vi "Autonomous Independent.vi"() -> ()   [LabVIEW 2020]
doc: "This VI is called when autonomous begins, and will automatically be terminated when autonomous ends. You can carry out timed or sensor driven robot movement independently without needing to return to the caller."
uses:
  <vilib>/Rock Robotics/WPI/Solenoid/WPI_SolenoidValue.ctl
  <vilib>/Rock Robotics/WPI/Utilities/WPI_GetSetVariantRefNum.vi
  <vilib>/Rock Robotics/Network Tables/NT Read String.vi
  <vilib>/Rock Robotics/Network Tables/NT Write Numeric Array.vi
  <vilib>/Rock Robotics/WPI/Solenoid/WPI_SolenoidSetEnum.vi
panel:
  out "substring":string
  in  "Array of robot movements 2":T1(array[cluster])=[{"X Joystick Value"=0.39393939393939403, "Y Joystick Value"=0.0, "Delay (sec)"=1.0, "Movement Name"="turn"}, {"X Joystick Value"=-0.3737373737373737, "Y Joystick Value"=0.0, "Delay (sec)"=1.0, "Movement Name"="turn back"}] {"Y Joystick Value" scale=1.0..-1.0; "X Joystick Value" scale=-1.0..1.0}
  # "Be sure to right-click and choose Data Operations>>Make Current Value default if you want to save the array values with the VI"
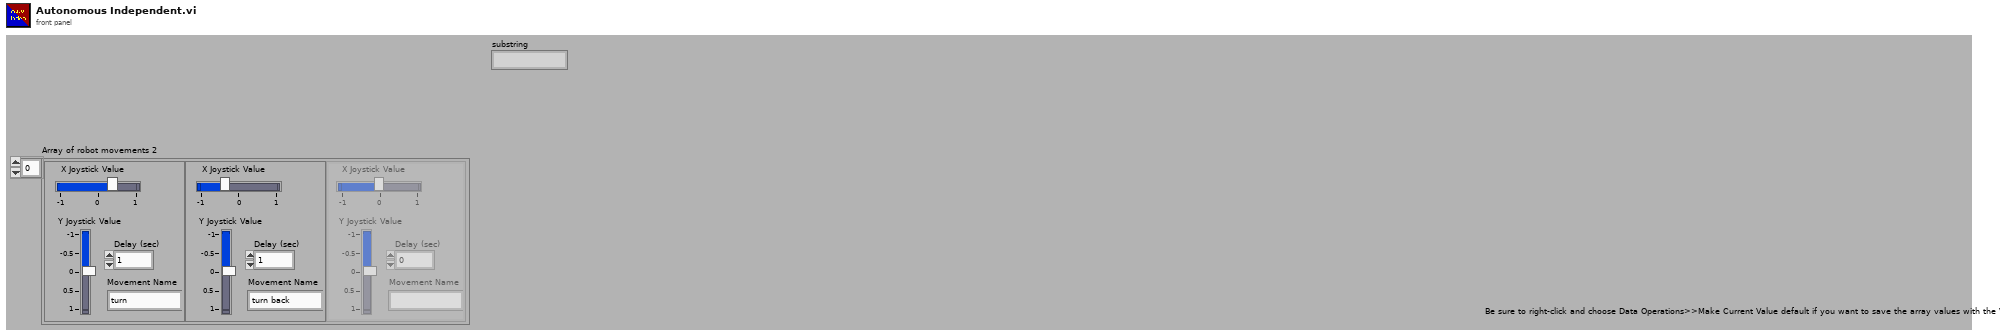
[diagram p1: front panel]
types:
  T1 = cluster{"X Joystick Value":dbl, "Y Joystick Value":dbl, "Delay (sec)":dbl, "Movement Name":string}[]
  T2 = typedef "WPI_JoystickDevRef.ctl" = cluster{"Device":T3}
  T3 = typedef "WPI_JoystickDeviceEnum.ctl" = enum16{"USB 0", "USB 1", "USB 2", "USB 3", "USB 4", "USB 5"}
  T4 = typedef "WPI_SolenoidValue.ctl" = enum16{"Off", "On", "Forward", "Reverse"}
  T5 = typedef "WPI_RobotDriveDevRef.ctl" = cluster{"DevStatus":errorcluster, "Motors[]":T6[], "Square Inputs":bool, "Max Output":dbl}
  T6 = typedef "WPI_MotorControlDeviceRef.ctl" = cluster{"DeviceStatus":errorcluster, "Type":T7, "PWM":cluster{"PWM Channel":T8, "DeadBand":T9}, "CAN":cluster{"Device Number":u8, "SetOutput VI Ref":variant, "GetOutput VI Ref":variant, "Enable VI Ref":variant, "Disable VI Ref":variant, "Data":variant}, "Invert":bool, "DIO PWM":cluster{"PWM \"Enable\" Channel":T8, "DIOChannel":T10, "PWM Rate":dbl}}
  T7 = typedef "WPI_MotorControlType.ctl" = enum16{"PWM", "CAN", "DIO PWM"}
  T8 = typedef "FPGA_DIOPWMChannel.ctl" = enum8{"PWM 0", "PWM 1", "PWM 2", "PWM 3", "PWM 4", "PWM 5", "PWM 6", "PWM 7", "PWM 8", "PWM 9", "PWM MXP 0", "PWM MXP 1", "PWM MXP 2", "PWM MXP 3", "PWM MXP 4", "PWM MXP 5", "PWM MXP 6", "PWM MXP 7", "PWM MXP 8", "PWM MXP 9", "Invalid"}
  T9 = typedef "WPI_PWMDeadband.ctl" = cluster{"Name":string, "maxPositivePwm":i32, "minPositivePwm":i32, "centerPwm":i32, "maxNegativePwm":i32, "minNegativePwm":i32, "angularRange":u16}
  T10 = typedef "FPGA_DIOChannel.ctl" = enum8{"DIO 0", "DIO 1", "DIO 2", "DIO 3", "DIO 4", "DIO 5", "DIO 6", "DIO 7", "DIO 8", "DIO 9", "DIO MXP 0", "DIO MXP 1", "DIO MXP 2", "DIO MXP 3", "DIO MXP 4", "DIO MXP 5", "DIO MXP 6", "DIO MXP 7", "DIO MXP 8", "DIO MXP 9", "DIO MXP 10", "DIO MXP 11", "DIO MXP 12", "DIO MXP 13", "DIO MXP 14", "DIO MXP 15", "SPI Port CS1", "SPI Port CS2", "SPI Port CS3", "SPI Port MISO", "SPI Port MOSI", "Invalid"}
  T11 = typedef "WPI_SolenoidDevRef.ctl" = cluster{"DevStatus":errorcluster, "Pneumatics Control Module":u8, "Forward Solenoid Channel":T12, "Reverse Solenoid Channel":T12}
  T12 = typedef "WPI_SolenoidChannel.ctl" = enum8{"Solenoid 0", "Solenoid 1", "Solenoid 2", "Solenoid 3", "Solenoid 4", "Solenoid 5", "Solenoid 6", "Solenoid 7", "Solenoid 8", "Solenoid 9", "Solenoid 10", "Solenoid 11", "Solenoid 12", "Solenoid 13", "Solenoid 14", "Solenoid 15", "Invalid"}
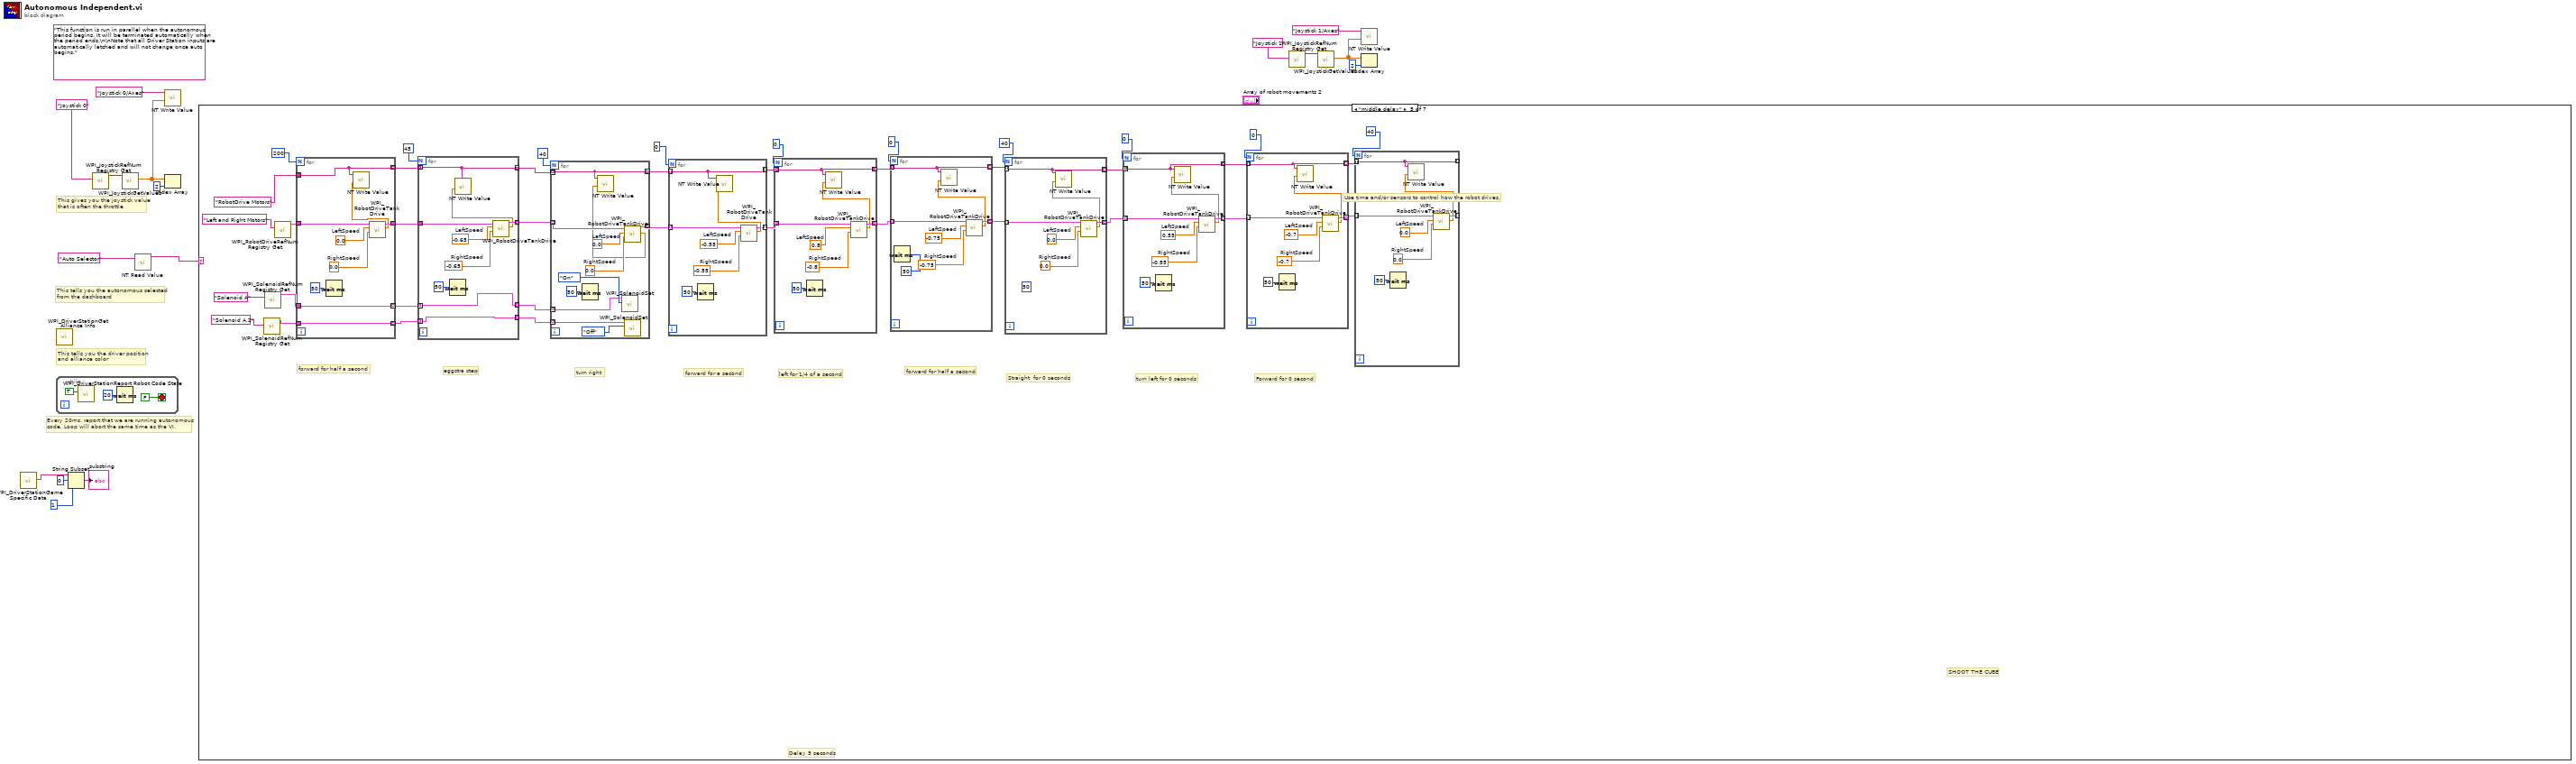
[diagram p0: block diagram]
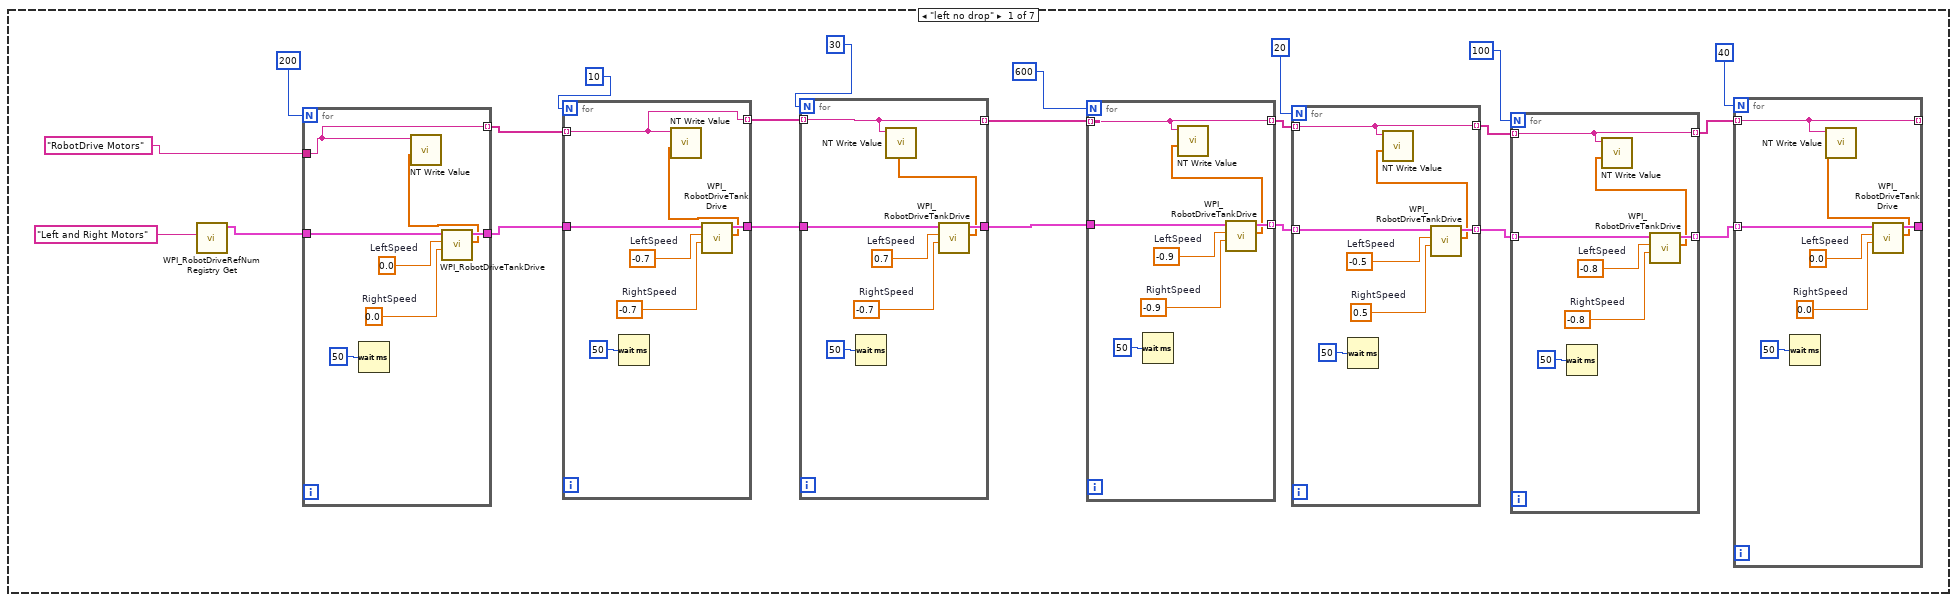
[diagram p2: hidden frame]
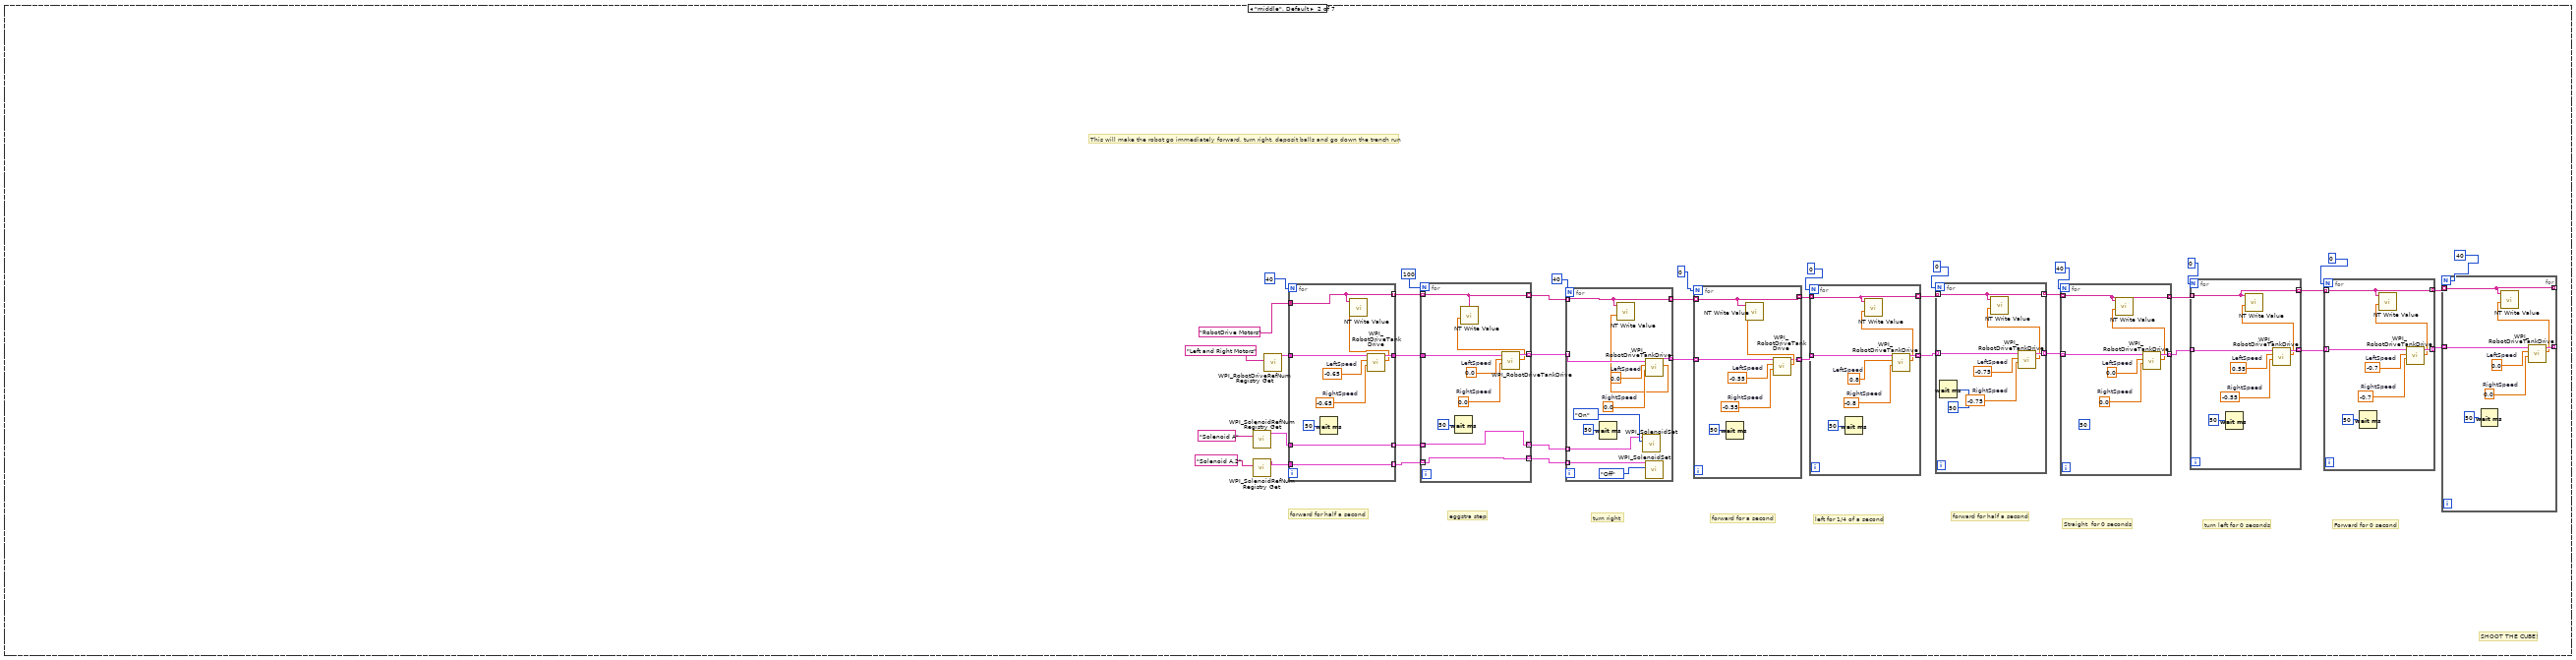
[diagram p3: hidden frame]
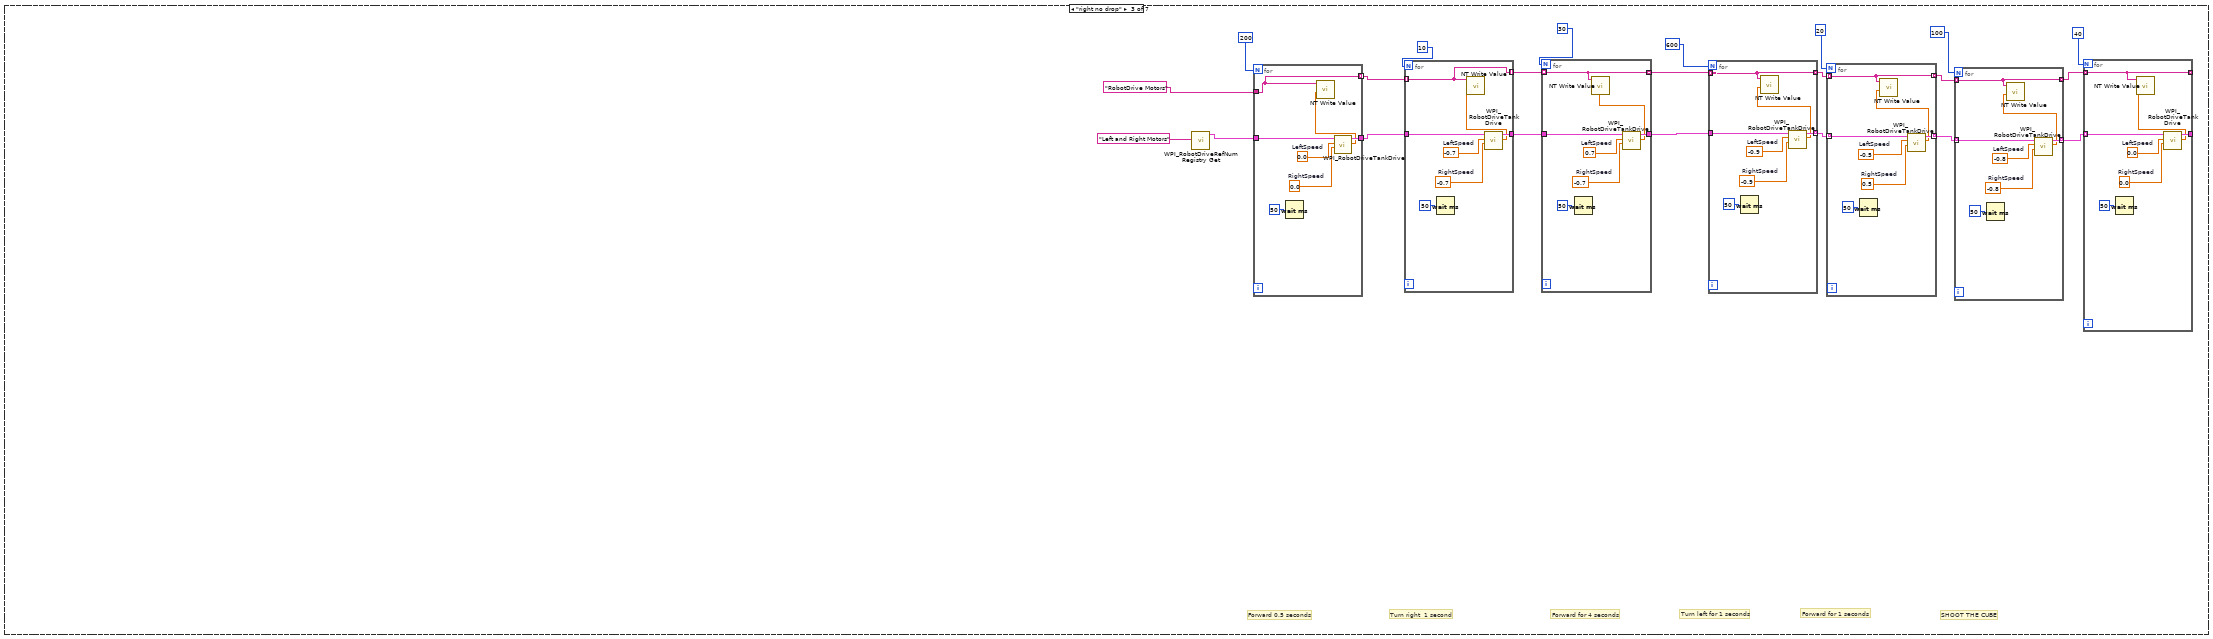
[diagram p4: hidden frame]
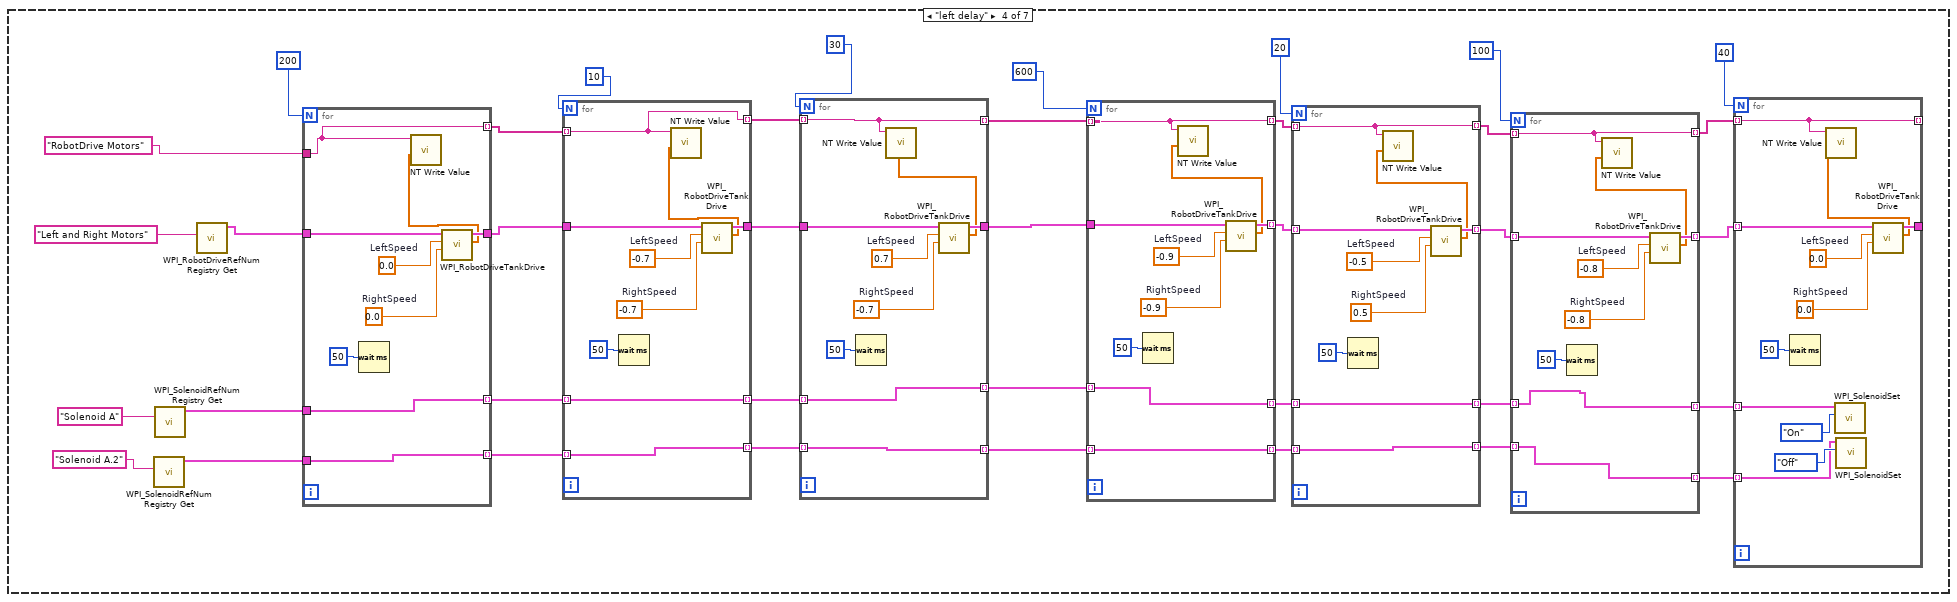
[diagram p5: hidden frame]
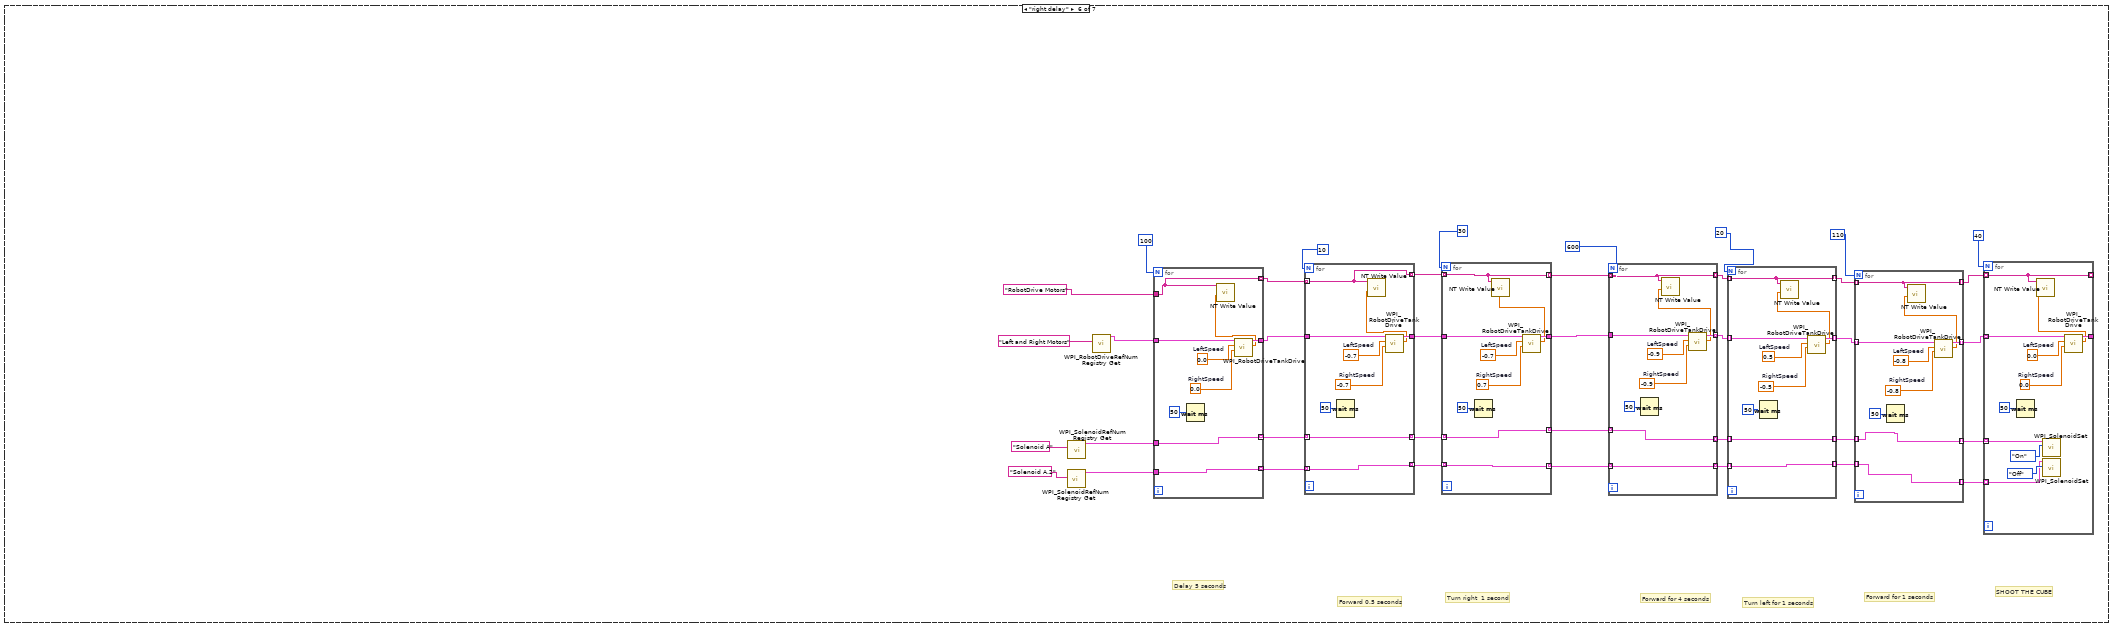
[diagram p6: hidden frame]
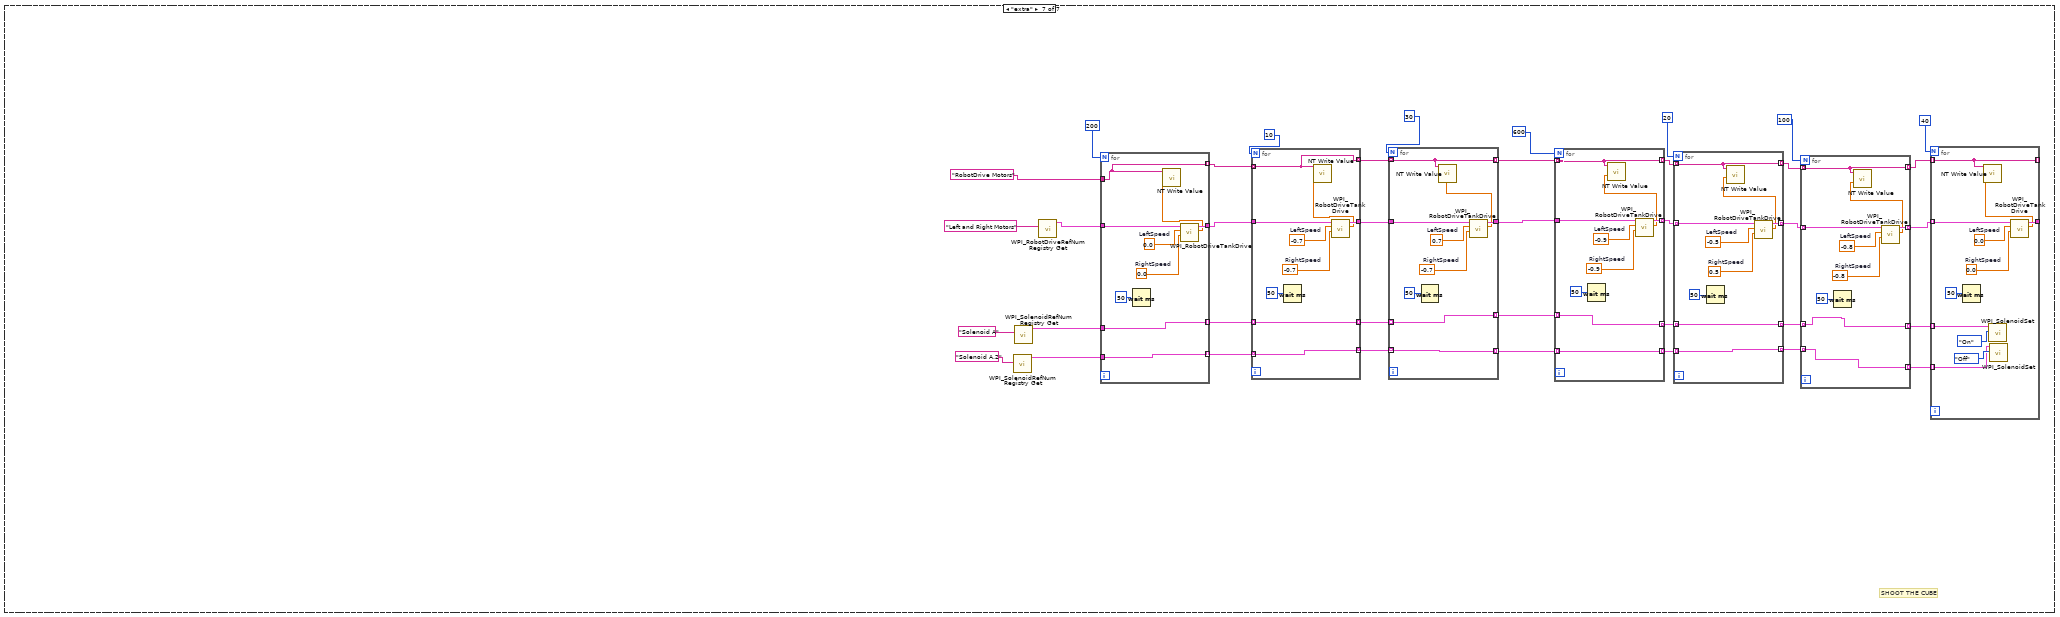
[diagram p7: hidden frame]
diagram:
  (unwired) "This function is run in parallel when the autonomous period begins. It will be terminated automatically when the period ends.\n\nNote that all Driver Station inputs are automatically latched and will not change once auto begins."
  # "This tells you the autonomous selected\nfrom the dashboard"
  # "Every 20ms, report that we are running autonomous\ncode. Loop will abort the same time as the VI."
  # "This gives you the joystick value\nthat is often the throttle"
  # "Use time and/or sensors to control how the robot drives."
  # "This tells you the driver position\nand alliance color"
  n1 = call <vilib>:"WPI_DriverStationGame Specific Data.vi"() -> ("Game Specific Data"=w4:string)  [unwired: 11 in]
  n2 = while {
    stop <- FALSE stop-if-true
    n3 = call <vilib>:"WPI_DriverStationReport Robot Code State.vi"("Autonomous"=TRUE) -> ()  [unwired: 10 in, 1 out]
    n4 = Wait (ms)(milliseconds to wait=u32 20) -> ()  [unwired: 1 out]
  }
  n5 = call <vilib>:"WPI_DriverStationGet Alliance Info.vi"() -> ()  [unwired: 12 out]
  n6 = String Subset(string=w4, offset (0)=0, length (rest)=1 ("length (rest)")) -> (substring=→"substring":string)
  n7 = call <vilib>:"WPI_JoystickRefNum Registry Get.vi"("refnum name"="Joystick 0") -> ("JoystickDevRef"=w15:T2)  [unwired: 1 in, 9 out]
  n8 = call <vilib>:"WPI_JoystickGetValues.vi"("JoystickDevRef"=w15) -> ("Axes"=w11:dbl[])  [unwired: 6 in, 4 out]
  n9 = call-poly <vilib>:"NT Read Value.vi"("Name"="Auto Selector") -> ("String"=w12:string)  [unwired: 9 in, 1 out]
  n10 = call-poly <vilib>:"NT Write Value.vi"("Numeric Array"=w11, "Name"="Joystick 0/Axes") -> ()  [unwired: 9 in, 1 out]
  n11 = Index Array(array=w11, index=2) -> ()  [unwired: 1 out]
  n12 = case shown="\"middle delay\"" w12 {
    frame "left no drop" {
      n13 = call <vilib>:"WPI_RobotDriveRefNum Registry Get.vi"("refnum name"="Left and Right Motors") -> ("RobotDriveDevRef"=w30:T5)  [unwired: 1 in, 9 out]
      n14 = for {
        N: 200 -> [_]
        tunnel: w30 -> [w48]
        tunnel: [w44] -> w29
        tunnel: [w42] -> w31 mode=indexing
        tunnel: "RobotDrive Motors" ("Name") -> [w42]
        w45 = 0.0  # RightSpeed
        w46 = 0.0  # LeftSpeed
        n15 = Wait (ms)(milliseconds to wait=u32 50) -> ()  [unwired: 1 out]
        n16 = call <vilib>:"WPI_RobotDriveTankDrive.vi"("Right axis value"=w45, "Left axis value"=w46, "RobotDriveDevRef"=w48) -> ("Motor Values"=w43:dbl[], "RobotDriveDevRef"=w44:T5)  [unwired: 6 in, 1 out]
        n17 = call-poly <vilib>:"NT Write Value.vi"("Numeric Array"=w43, "Name"=w42) -> ()  [unwired: 9 in, 1 out]
      }
      n18 = for {
        N: 10 -> [_]
        tunnel: w29 -> [w90]
        tunnel: [w86] -> w41
        tunnel: [w84] -> w40 mode=indexing
        tunnel: w31 -> [w84] mode=indexing
        w87 = -0.7  # RightSpeed
        w88 = -0.7  # LeftSpeed
        n19 = Wait (ms)(milliseconds to wait=u32 50) -> ()  [unwired: 1 out]
        n20 = call <vilib>:"WPI_RobotDriveTankDrive.vi"("Right axis value"=w87, "Left axis value"=w88, "RobotDriveDevRef"=w90) -> ("Motor Values"=w85:dbl[], "RobotDriveDevRef"=w86:T5)  [unwired: 6 in, 1 out]
        n21 = call-poly <vilib>:"NT Write Value.vi"("Numeric Array"=w85, "Name"=w84) -> ()  [unwired: 9 in, 1 out]
      }
      n22 = for {
        N: 30 -> [_]
        tunnel: w41 -> [w76]
        tunnel: [w72] -> w38
        tunnel: [w70] -> w39 mode=indexing
        tunnel: w40 -> [w70] mode=indexing
        w73 = -0.7  # RightSpeed
        w74 = 0.7  # LeftSpeed
        n23 = Wait (ms)(milliseconds to wait=u32 50) -> ()  [unwired: 1 out]
        n24 = call <vilib>:"WPI_RobotDriveTankDrive.vi"("Right axis value"=w73, "Left axis value"=w74, "RobotDriveDevRef"=w76) -> ("Motor Values"=w71:dbl[], "RobotDriveDevRef"=w72:T5)  [unwired: 6 in, 1 out]
        n25 = call-poly <vilib>:"NT Write Value.vi"("Numeric Array"=w71, "Name"=w70) -> ()  [unwired: 9 in, 1 out]
      }
      n26 = for {
        N: 600 -> [_]
        tunnel: w38 -> [w69]
        tunnel: [w65] -> w34 mode=indexing
        tunnel: w39 -> [w63] mode=indexing
        tunnel: [w63] -> w37 mode=indexing
        w66 = -0.9  # RightSpeed
        w67 = -0.9  # LeftSpeed
        n27 = Wait (ms)(milliseconds to wait=u32 50) -> ()  [unwired: 1 out]
        n28 = call <vilib>:"WPI_RobotDriveTankDrive.vi"("Right axis value"=w66, "Left axis value"=w67, "RobotDriveDevRef"=w69) -> ("Motor Values"=w64:dbl[], "RobotDriveDevRef"=w65:T5)  [unwired: 6 in, 1 out]
        n29 = call-poly <vilib>:"NT Write Value.vi"("Numeric Array"=w64, "Name"=w63) -> ()  [unwired: 9 in, 1 out]
      }
      n30 = for {
        N: 20 -> [_]
        tunnel: w34 -> [w62] mode=indexing
        tunnel: [w58] -> w33 mode=indexing
        tunnel: w37 -> [w56] mode=indexing
        tunnel: [w56] -> w36 mode=indexing
        w59 = 0.5  # RightSpeed
        w60 = -0.5  # LeftSpeed
        n31 = Wait (ms)(milliseconds to wait=u32 50) -> ()  [unwired: 1 out]
        n32 = call <vilib>:"WPI_RobotDriveTankDrive.vi"("Right axis value"=w59, "Left axis value"=w60, "RobotDriveDevRef"=w62) -> ("Motor Values"=w57:dbl[], "RobotDriveDevRef"=w58:T5)  [unwired: 6 in, 1 out]
        n33 = call-poly <vilib>:"NT Write Value.vi"("Numeric Array"=w57, "Name"=w56) -> ()  [unwired: 9 in, 1 out]
      }
      n34 = for {
        N: 100 -> [_]
        tunnel: w33 -> [w55] mode=indexing
        tunnel: [w51] -> w32 mode=indexing
        tunnel: w36 -> [w49] mode=indexing
        tunnel: [w49] -> w35 mode=indexing
        w52 = -0.8  # RightSpeed
        w53 = -0.8  # LeftSpeed
        n35 = Wait (ms)(milliseconds to wait=u32 50) -> ()  [unwired: 1 out]
        n36 = call <vilib>:"WPI_RobotDriveTankDrive.vi"("Right axis value"=w52, "Left axis value"=w53, "RobotDriveDevRef"=w55) -> ("Motor Values"=w50:dbl[], "RobotDriveDevRef"=w51:T5)  [unwired: 6 in, 1 out]
        n37 = call-poly <vilib>:"NT Write Value.vi"("Numeric Array"=w50, "Name"=w49) -> ()  [unwired: 9 in, 1 out]
      }
      n38 = for {
        N: 40 -> [_]
        tunnel: w32 -> [w83] mode=indexing
        tunnel: [w79] -> _
        tunnel: [w77] -> _ mode=indexing
        tunnel: w35 -> [w77] mode=indexing
        w80 = 0.0  # RightSpeed
        w81 = 0.0  # LeftSpeed
        n39 = Wait (ms)(milliseconds to wait=u32 50) -> ()  [unwired: 1 out]
        n40 = call <vilib>:"WPI_RobotDriveTankDrive.vi"("Right axis value"=w80, "Left axis value"=w81, "RobotDriveDevRef"=w83) -> ("Motor Values"=w78:dbl[], "RobotDriveDevRef"=w79:T5)  [unwired: 6 in, 1 out]
        n41 = call-poly <vilib>:"NT Write Value.vi"("Numeric Array"=w78, "Name"=w77) -> ()  [unwired: 9 in, 1 out]
      }
    }
    frame "middle", Default {
      # "SHOOT THE CUBE!"
      # "Forward for 0 second"
      # "turn left for 0 seconds"
      # "Straight  for 0 seconds"
      # "forward for half a second"
      # "turn right"
      # "left for 1/4 of a second"
      # "forward for a second"
      # "eggstra step"
      # "forward for half a second"
      # "This will make the robot go immediately forward, turn right, deposit balls and go down the trench run"
      n42 = call <vilib>:"WPI_SolenoidRefNum Registry Get.vi"("refnum name"="Solenoid A.2") -> ("SolenoidDevRef"=w96:T11)  [unwired: 9 in, 1 out]
      n43 = call <vilib>:"WPI_SolenoidRefNum Registry Get.vi"("refnum name"="Solenoid A") -> ("SolenoidDevRef"=w98:T11)  [unwired: 9 in, 1 out]
      n44 = call <vilib>:"WPI_RobotDriveRefNum Registry Get.vi"("refnum name"="Left and Right Motors") -> ("RobotDriveDevRef"=w128:T5)  [unwired: 1 in, 9 out]
      n45 = for {
        N: 40 -> [_]
        tunnel: w128 -> [w206]
        tunnel: [w202] -> w126
        tunnel: "RobotDrive Motors" ("Name") -> [w200]
        tunnel: [w200] -> w124 mode=indexing
        tunnel: w98 -> [w199]
        tunnel: [w199] -> w97 mode=indexing
        tunnel: w96 -> [w198]
        tunnel: [w198] -> w95 mode=indexing
        w203 = -0.65  # RightSpeed
        w204 = -0.65  # LeftSpeed
        n46 = Wait (ms)(milliseconds to wait=u32 50) -> ()  [unwired: 1 out]
        n47 = call <vilib>:"WPI_RobotDriveTankDrive.vi"("Right axis value"=w203, "Left axis value"=w204, "RobotDriveDevRef"=w206) -> ("Motor Values"=w201:dbl[], "RobotDriveDevRef"=w202:T5)  [unwired: 6 in, 1 out]
        n48 = call-poly <vilib>:"NT Write Value.vi"("Numeric Array"=w201, "Name"=w200) -> ()  [unwired: 9 in, 1 out]
      }
      n49 = for {
        N: 100 -> [_]
        tunnel: w126 -> [w190]
        tunnel: [w194] -> w120 mode=indexing
        tunnel: w124 -> [w194] mode=indexing
        tunnel: w97 -> [w191] mode=indexing
        tunnel: w95 -> [w192] mode=indexing
        tunnel: [w191] -> w93 mode=indexing
        tunnel: [w192] -> w92 mode=indexing
        tunnel: [w193] -> w91 mode=indexing
        w195 = 0.0  # RightSpeed
        w196 = 0.0  # LeftSpeed
        n50 = Wait (ms)(milliseconds to wait=u32 50) -> ()  [unwired: 1 out]
        n51 = call <vilib>:"WPI_RobotDriveTankDrive.vi"("Right axis value"=w195, "Left axis value"=w196, "RobotDriveDevRef"=w190) -> ("Motor Values"=w189:dbl[], "RobotDriveDevRef"=w193:T5)  [unwired: 6 in, 1 out]
        n52 = call-poly <vilib>:"NT Write Value.vi"("Numeric Array"=w189, "Name"=w194) -> ()  [unwired: 9 in, 1 out]
      }
      n53 = for {
        N: 40 -> [_]
        tunnel: [w165] -> w121 mode=indexing
        tunnel: w120 -> [w166] mode=indexing
        tunnel: [w166] -> w122 mode=indexing
        tunnel: w93 -> [w167] mode=indexing
        tunnel: w92 -> [w169] mode=indexing
        tunnel: w91 -> [w168] mode=indexing
        w172 = 0.0  # RightSpeed
        w173 = 0.0  # LeftSpeed
        n54 = Wait (ms)(milliseconds to wait=u32 50) -> ()  [unwired: 1 out]
        n55 = call-poly <vilib>:"WPI_SolenoidSet.vi"("Value"=WPI_SolenoidValue."On", "SolenoidDevRef"=w167) -> ()  [unwired: 8 in, 2 out]
        n56 = call <vilib>:"WPI_RobotDriveTankDrive.vi"("Right axis value"=w172, "Left axis value"=w173, "RobotDriveDevRef"=w168) -> ("Motor Values"=w164:dbl[], "RobotDriveDevRef"=w165:T5)  [unwired: 6 in, 1 out]
        n57 = call-poly <vilib>:"NT Write Value.vi"("Numeric Array"=w164, "Name"=w166) -> ()  [unwired: 9 in, 1 out]
        n58 = call-poly <vilib>:"WPI_SolenoidSet.vi"("Value"=WPI_SolenoidValue."Off", "SolenoidDevRef"=w169) -> ()  [unwired: 8 in, 2 out]
      }
      n59 = for {
        N: 0 -> [_]
        tunnel: w121 -> [w188] mode=indexing
        tunnel: w122 -> [w183] mode=indexing
        tunnel: [w183] -> w119 mode=indexing
        tunnel: [w182] -> w118 mode=indexing
        w185 = -0.55  # RightSpeed
        w186 = -0.55  # LeftSpeed
        n60 = Wait (ms)(milliseconds to wait=u32 50) -> ()  [unwired: 1 out]
        n61 = call <vilib>:"WPI_RobotDriveTankDrive.vi"("Right axis value"=w185, "Left axis value"=w186, "RobotDriveDevRef"=w188) -> ("Motor Values"=w184:dbl[], "RobotDriveDevRef"=w182:T5)  [unwired: 6 in, 1 out]
        n62 = call-poly <vilib>:"NT Write Value.vi"("Numeric Array"=w184, "Name"=w183) -> ()  [unwired: 9 in, 1 out]
      }
      n63 = for {
        N: 0 -> [_]
        tunnel: w118 -> [w181] mode=indexing
        tunnel: [w178] -> w113 mode=indexing
        tunnel: w119 -> [w176] mode=indexing
        tunnel: [w176] -> w114 mode=indexing
        w175 = 0.8  # LeftSpeed
        w179 = -0.8  # RightSpeed
        n64 = Wait (ms)(milliseconds to wait=u32 50) -> ()  [unwired: 1 out]
        n65 = call <vilib>:"WPI_RobotDriveTankDrive.vi"("Right axis value"=w179, "Left axis value"=w175, "RobotDriveDevRef"=w181) -> ("Motor Values"=w177:dbl[], "RobotDriveDevRef"=w178:T5)  [unwired: 6 in, 1 out]
        n66 = call-poly <vilib>:"NT Write Value.vi"("Numeric Array"=w177, "Name"=w176) -> ()  [unwired: 9 in, 1 out]
      }
      n67 = for {
        N: 0 -> [_]
        tunnel: w113 -> [w163] mode=indexing
        tunnel: [w159] -> w110 mode=indexing
        tunnel: w114 -> [w157] mode=indexing
        tunnel: [w157] -> w111 mode=indexing
        w160 = -0.75  # RightSpeed
        w161 = -0.75  # LeftSpeed
        n68 = Wait (ms)(milliseconds to wait=u32 50) -> ()  [unwired: 1 out]
        n69 = call <vilib>:"WPI_RobotDriveTankDrive.vi"("Right axis value"=w160, "Left axis value"=w161, "RobotDriveDevRef"=w163) -> ("Motor Values"=w158:dbl[], "RobotDriveDevRef"=w159:T5)  [unwired: 6 in, 1 out]
        n70 = call-poly <vilib>:"NT Write Value.vi"("Numeric Array"=w158, "Name"=w157) -> ()  [unwired: 9 in, 1 out]
      }
      n71 = for {
        N: 40 -> [_]
        tunnel: w110 -> [w156] mode=indexing
        tunnel: [w153] -> w107 mode=indexing
        tunnel: w111 -> [w151] mode=indexing
        tunnel: [w151] -> w108 mode=indexing
        w154 = 0.0  # RightSpeed
        w155 = 0.0  # LeftSpeed
        (unwired) u32 50 ("milliseconds to wait")
        n72 = call <vilib>:"WPI_RobotDriveTankDrive.vi"("Right axis value"=w154, "Left axis value"=w155, "RobotDriveDevRef"=w156) -> ("Motor Values"=w152:dbl[], "RobotDriveDevRef"=w153:T5)  [unwired: 6 in, 1 out]
        n73 = call-poly <vilib>:"NT Write Value.vi"("Numeric Array"=w152, "Name"=w151) -> ()  [unwired: 9 in, 1 out]
      }
      n74 = for {
        N: 0 -> [_]
        tunnel: w107 -> [w150] mode=indexing
        tunnel: [w146] -> w104 mode=indexing
        tunnel: w108 -> [w144] mode=indexing
        tunnel: [w144] -> w105 mode=indexing
        w147 = -0.55  # RightSpeed
        w148 = 0.55  # LeftSpeed
        n75 = Wait (ms)(milliseconds to wait=u32 50) -> ()  [unwired: 1 out]
        n76 = call <vilib>:"WPI_RobotDriveTankDrive.vi"("Right axis value"=w147, "Left axis value"=w148, "RobotDriveDevRef"=w150) -> ("Motor Values"=w145:dbl[], "RobotDriveDevRef"=w146:T5)  [unwired: 6 in, 1 out]
        n77 = call-poly <vilib>:"NT Write Value.vi"("Numeric Array"=w145, "Name"=w144) -> ()  [unwired: 9 in, 1 out]
      }
      n78 = for {
        N: 0 -> [_]
        tunnel: w104 -> [w143] mode=indexing
        tunnel: [w139] -> w103 mode=indexing
        tunnel: w105 -> [w137] mode=indexing
        tunnel: [w137] -> w102 mode=indexing
        w140 = -0.7  # RightSpeed
        w141 = -0.7  # LeftSpeed
        n79 = Wait (ms)(milliseconds to wait=u32 50) -> ()  [unwired: 1 out]
        n80 = call <vilib>:"WPI_RobotDriveTankDrive.vi"("Right axis value"=w140, "Left axis value"=w141, "RobotDriveDevRef"=w143) -> ("Motor Values"=w138:dbl[], "RobotDriveDevRef"=w139:T5)  [unwired: 6 in, 1 out]
        n81 = call-poly <vilib>:"NT Write Value.vi"("Numeric Array"=w138, "Name"=w137) -> ()  [unwired: 9 in, 1 out]
      }
      n82 = for {
        N: 40 -> [_]
        tunnel: w103 -> [w136] mode=indexing
        tunnel: [w132] -> _ mode=indexing
        tunnel: w102 -> [w130] mode=indexing
        tunnel: [w130] -> _ mode=indexing
        w133 = 0.0  # RightSpeed
        w134 = 0.0  # LeftSpeed
        n83 = Wait (ms)(milliseconds to wait=u32 50) -> ()  [unwired: 1 out]
        n84 = call <vilib>:"WPI_RobotDriveTankDrive.vi"("Right axis value"=w133, "Left axis value"=w134, "RobotDriveDevRef"=w136) -> ("Motor Values"=w131:dbl[], "RobotDriveDevRef"=w132:T5)  [unwired: 6 in, 1 out]
        n85 = call-poly <vilib>:"NT Write Value.vi"("Numeric Array"=w131, "Name"=w130) -> ()  [unwired: 9 in, 1 out]
      }
    }
    frame "right no drop" {
      # "Forward for 1 seconds"
      # "Turn left for 1 seconds"
      # "Forward for 4 seconds"
      # "Turn right  1 second"
      # "SHOOT THE CUBE"
      # "Forward 0.5 seconds"
      n86 = call <vilib>:"WPI_RobotDriveRefNum Registry Get.vi"("refnum name"="Left and Right Motors") -> ("RobotDriveDevRef"=w227:T5)  [unwired: 1 in, 9 out]
      n87 = for {
        N: 200 -> [_]
        tunnel: w227 -> [w235]
        tunnel: [w231] -> w228
        tunnel: [w229] -> w226 mode=indexing
        tunnel: "RobotDrive Motors" ("Name") -> [w229]
        w232 = 0.0  # RightSpeed
        w233 = 0.0  # LeftSpeed
        n88 = Wait (ms)(milliseconds to wait=u32 50) -> ()  [unwired: 1 out]
        n89 = call <vilib>:"WPI_RobotDriveTankDrive.vi"("Right axis value"=w232, "Left axis value"=w233, "RobotDriveDevRef"=w235) -> ("Motor Values"=w230:dbl[], "RobotDriveDevRef"=w231:T5)  [unwired: 6 in, 1 out]
        n90 = call-poly <vilib>:"NT Write Value.vi"("Numeric Array"=w230, "Name"=w229) -> ()  [unwired: 9 in, 1 out]
      }
      n91 = for {
        N: 10 -> [_]
        tunnel: w228 -> [w277]
        tunnel: [w273] -> w216
        tunnel: [w271] -> w217 mode=indexing
        tunnel: w226 -> [w271] mode=indexing
        w274 = -0.7  # RightSpeed
        w275 = -0.7  # LeftSpeed
        n92 = Wait (ms)(milliseconds to wait=u32 50) -> ()  [unwired: 1 out]
        n93 = call <vilib>:"WPI_RobotDriveTankDrive.vi"("Right axis value"=w274, "Left axis value"=w275, "RobotDriveDevRef"=w277) -> ("Motor Values"=w272:dbl[], "RobotDriveDevRef"=w273:T5)  [unwired: 6 in, 1 out]
        n94 = call-poly <vilib>:"NT Write Value.vi"("Numeric Array"=w272, "Name"=w271) -> ()  [unwired: 9 in, 1 out]
      }
      n95 = for {
        N: 30 -> [_]
        tunnel: w216 -> [w263]
        tunnel: [w259] -> w219
        tunnel: [w257] -> w218 mode=indexing
        tunnel: w217 -> [w257] mode=indexing
        w260 = -0.7  # RightSpeed
        w261 = 0.7  # LeftSpeed
        n96 = Wait (ms)(milliseconds to wait=u32 50) -> ()  [unwired: 1 out]
        n97 = call <vilib>:"WPI_RobotDriveTankDrive.vi"("Right axis value"=w260, "Left axis value"=w261, "RobotDriveDevRef"=w263) -> ("Motor Values"=w258:dbl[], "RobotDriveDevRef"=w259:T5)  [unwired: 6 in, 1 out]
        n98 = call-poly <vilib>:"NT Write Value.vi"("Numeric Array"=w258, "Name"=w257) -> ()  [unwired: 9 in, 1 out]
      }
      n99 = for {
        N: 600 -> [_]
        tunnel: w219 -> [w256]
        tunnel: [w252] -> w223 mode=indexing
        tunnel: w218 -> [w250] mode=indexing
        tunnel: [w250] -> w220 mode=indexing
        w253 = -0.9  # RightSpeed
        w254 = -0.9  # LeftSpeed
        n100 = Wait (ms)(milliseconds to wait=u32 50) -> ()  [unwired: 1 out]
        n101 = call <vilib>:"WPI_RobotDriveTankDrive.vi"("Right axis value"=w253, "Left axis value"=w254, "RobotDriveDevRef"=w256) -> ("Motor Values"=w251:dbl[], "RobotDriveDevRef"=w252:T5)  [unwired: 6 in, 1 out]
        n102 = call-poly <vilib>:"NT Write Value.vi"("Numeric Array"=w251, "Name"=w250) -> ()  [unwired: 9 in, 1 out]
      }
      n103 = for {
        N: 20 -> [_]
        tunnel: w223 -> [w249] mode=indexing
        tunnel: [w245] -> w224 mode=indexing
        tunnel: w220 -> [w243] mode=indexing
        tunnel: [w243] -> w221 mode=indexing
        w246 = 0.5  # RightSpeed
        w247 = -0.5  # LeftSpeed
        n104 = Wait (ms)(milliseconds to wait=u32 50) -> ()  [unwired: 1 out]
        n105 = call <vilib>:"WPI_RobotDriveTankDrive.vi"("Right axis value"=w246, "Left axis value"=w247, "RobotDriveDevRef"=w249) -> ("Motor Values"=w244:dbl[], "RobotDriveDevRef"=w245:T5)  [unwired: 6 in, 1 out]
        n106 = call-poly <vilib>:"NT Write Value.vi"("Numeric Array"=w244, "Name"=w243) -> ()  [unwired: 9 in, 1 out]
      }
      n107 = for {
        N: 100 -> [_]
        tunnel: w224 -> [w242] mode=indexing
        tunnel: [w238] -> w225 mode=indexing
        tunnel: w221 -> [w236] mode=indexing
        tunnel: [w236] -> w222 mode=indexing
        w239 = -0.8  # RightSpeed
        w240 = -0.8  # LeftSpeed
        n108 = Wait (ms)(milliseconds to wait=u32 50) -> ()  [unwired: 1 out]
        n109 = call <vilib>:"WPI_RobotDriveTankDrive.vi"("Right axis value"=w239, "Left axis value"=w240, "RobotDriveDevRef"=w242) -> ("Motor Values"=w237:dbl[], "RobotDriveDevRef"=w238:T5)  [unwired: 6 in, 1 out]
        n110 = call-poly <vilib>:"NT Write Value.vi"("Numeric Array"=w237, "Name"=w236) -> ()  [unwired: 9 in, 1 out]
      }
      n111 = for {
        N: 40 -> [_]
        tunnel: w225 -> [w270] mode=indexing
        tunnel: [w266] -> _
        tunnel: [w264] -> _ mode=indexing
        tunnel: w222 -> [w264] mode=indexing
        w267 = 0.0  # RightSpeed
        w268 = 0.0  # LeftSpeed
        n112 = Wait (ms)(milliseconds to wait=u32 50) -> ()  [unwired: 1 out]
        n113 = call <vilib>:"WPI_RobotDriveTankDrive.vi"("Right axis value"=w267, "Left axis value"=w268, "RobotDriveDevRef"=w270) -> ("Motor Values"=w265:dbl[], "RobotDriveDevRef"=w266:T5)  [unwired: 6 in, 1 out]
        n114 = call-poly <vilib>:"NT Write Value.vi"("Numeric Array"=w265, "Name"=w264) -> ()  [unwired: 9 in, 1 out]
      }
    }
    frame "left delay" {
      n115 = call <vilib>:"WPI_SolenoidRefNum Registry Get.vi"("refnum name"="Solenoid A.2") -> ("SolenoidDevRef"=w291:T11)  [unwired: 9 in, 1 out]
      n116 = call <vilib>:"WPI_SolenoidRefNum Registry Get.vi"("refnum name"="Solenoid A") -> ("SolenoidDevRef"=w297:T11)  [unwired: 9 in, 1 out]
      n117 = call <vilib>:"WPI_RobotDriveRefNum Registry Get.vi"("refnum name"="Left and Right Motors") -> ("RobotDriveDevRef"=w304:T5)  [unwired: 1 in, 9 out]
      n118 = for {
        N: 200 -> [_]
        tunnel: w304 -> [w324]
        tunnel: [w320] -> w303
        tunnel: [w318] -> w305 mode=indexing
        tunnel: "RobotDrive Motors" ("Name") -> [w318]
        tunnel: [w317] -> w298 mode=indexing
        tunnel: w297 -> [w317]
        tunnel: [w316] -> w292 mode=indexing
        tunnel: w291 -> [w316]
        w321 = 0.0  # RightSpeed
        w322 = 0.0  # LeftSpeed
        n119 = Wait (ms)(milliseconds to wait=u32 50) -> ()  [unwired: 1 out]
        n120 = call <vilib>:"WPI_RobotDriveTankDrive.vi"("Right axis value"=w321, "Left axis value"=w322, "RobotDriveDevRef"=w324) -> ("Motor Values"=w319:dbl[], "RobotDriveDevRef"=w320:T5)  [unwired: 6 in, 1 out]
        n121 = call-poly <vilib>:"NT Write Value.vi"("Numeric Array"=w319, "Name"=w318) -> ()  [unwired: 9 in, 1 out]
      }
      n122 = for {
        N: 10 -> [_]
        tunnel: w303 -> [w380]
        tunnel: [w376] -> w315
        tunnel: [w374] -> w314 mode=indexing
        tunnel: w305 -> [w374] mode=indexing
        tunnel: [w373] -> w299 mode=indexing
        tunnel: w298 -> [w373] mode=indexing
        tunnel: [w372] -> w293 mode=indexing
        tunnel: w292 -> [w372] mode=indexing
        w377 = -0.7  # RightSpeed
        w378 = -0.7  # LeftSpeed
        n123 = Wait (ms)(milliseconds to wait=u32 50) -> ()  [unwired: 1 out]
        n124 = call <vilib>:"WPI_RobotDriveTankDrive.vi"("Right axis value"=w377, "Left axis value"=w378, "RobotDriveDevRef"=w380) -> ("Motor Values"=w375:dbl[], "RobotDriveDevRef"=w376:T5)  [unwired: 6 in, 1 out]
        n125 = call-poly <vilib>:"NT Write Value.vi"("Numeric Array"=w375, "Name"=w374) -> ()  [unwired: 9 in, 1 out]
      }
      n126 = for {
        N: 30 -> [_]
        tunnel: w315 -> [w360]
        tunnel: [w356] -> w312
        tunnel: [w354] -> w313 mode=indexing
        tunnel: w314 -> [w354] mode=indexing
        tunnel: [w353] -> w300 mode=indexing
        tunnel: w299 -> [w353] mode=indexing
        tunnel: [w352] -> w294 mode=indexing
        tunnel: w293 -> [w352] mode=indexing
        w357 = -0.7  # RightSpeed
        w358 = 0.7  # LeftSpeed
        n127 = Wait (ms)(milliseconds to wait=u32 50) -> ()  [unwired: 1 out]
        n128 = call <vilib>:"WPI_RobotDriveTankDrive.vi"("Right axis value"=w357, "Left axis value"=w358, "RobotDriveDevRef"=w360) -> ("Motor Values"=w355:dbl[], "RobotDriveDevRef"=w356:T5)  [unwired: 6 in, 1 out]
        n129 = call-poly <vilib>:"NT Write Value.vi"("Numeric Array"=w355, "Name"=w354) -> ()  [unwired: 9 in, 1 out]
      }
      n130 = for {
        N: 600 -> [_]
        tunnel: w312 -> [w351]
        tunnel: [w347] -> w308 mode=indexing
        tunnel: w313 -> [w345] mode=indexing
        tunnel: [w345] -> w311 mode=indexing
        tunnel: [w344] -> w301 mode=indexing
        tunnel: w300 -> [w344] mode=indexing
        tunnel: [w343] -> w295 mode=indexing
        tunnel: w294 -> [w343] mode=indexing
        w348 = -0.9  # RightSpeed
        w349 = -0.9  # LeftSpeed
        n131 = Wait (ms)(milliseconds to wait=u32 50) -> ()  [unwired: 1 out]
        n132 = call <vilib>:"WPI_RobotDriveTankDrive.vi"("Right axis value"=w348, "Left axis value"=w349, "RobotDriveDevRef"=w351) -> ("Motor Values"=w346:dbl[], "RobotDriveDevRef"=w347:T5)  [unwired: 6 in, 1 out]
        n133 = call-poly <vilib>:"NT Write Value.vi"("Numeric Array"=w346, "Name"=w345) -> ()  [unwired: 9 in, 1 out]
      }
      n134 = for {
        N: 20 -> [_]
        tunnel: w308 -> [w342] mode=indexing
        tunnel: [w338] -> w307 mode=indexing
        tunnel: w311 -> [w336] mode=indexing
        tunnel: [w336] -> w310 mode=indexing
        tunnel: [w335] -> w302 mode=indexing
        tunnel: w301 -> [w335] mode=indexing
        tunnel: [w334] -> w296 mode=indexing
        tunnel: w295 -> [w334] mode=indexing
        w339 = 0.5  # RightSpeed
        w340 = -0.5  # LeftSpeed
        n135 = Wait (ms)(milliseconds to wait=u32 50) -> ()  [unwired: 1 out]
        n136 = call <vilib>:"WPI_RobotDriveTankDrive.vi"("Right axis value"=w339, "Left axis value"=w340, "RobotDriveDevRef"=w342) -> ("Motor Values"=w337:dbl[], "RobotDriveDevRef"=w338:T5)  [unwired: 6 in, 1 out]
        n137 = call-poly <vilib>:"NT Write Value.vi"("Numeric Array"=w337, "Name"=w336) -> ()  [unwired: 9 in, 1 out]
      }
      n138 = for {
        N: 100 -> [_]
        tunnel: w307 -> [w333] mode=indexing
        tunnel: [w329] -> w306 mode=indexing
        tunnel: w310 -> [w327] mode=indexing
        tunnel: [w327] -> w309 mode=indexing
        tunnel: w302 -> [w326] mode=indexing
        tunnel: w296 -> [w325] mode=indexing
        tunnel: [w326] -> w290 mode=indexing
        tunnel: [w325] -> w289 mode=indexing
        w330 = -0.8  # RightSpeed
        w331 = -0.8  # LeftSpeed
        n139 = Wait (ms)(milliseconds to wait=u32 50) -> ()  [unwired: 1 out]
        n140 = call <vilib>:"WPI_RobotDriveTankDrive.vi"("Right axis value"=w330, "Left axis value"=w331, "RobotDriveDevRef"=w333) -> ("Motor Values"=w328:dbl[], "RobotDriveDevRef"=w329:T5)  [unwired: 6 in, 1 out]
        n141 = call-poly <vilib>:"NT Write Value.vi"("Numeric Array"=w328, "Name"=w327) -> ()  [unwired: 9 in, 1 out]
      }
      n142 = for {
        N: 40 -> [_]
        tunnel: w306 -> [w371] mode=indexing
        tunnel: [w367] -> _
        tunnel: [w365] -> _ mode=indexing
        tunnel: w309 -> [w365] mode=indexing
        tunnel: w290 -> [w362] mode=indexing
        tunnel: w289 -> [w361] mode=indexing
        w368 = 0.0  # RightSpeed
        w369 = 0.0  # LeftSpeed
        n143 = Wait (ms)(milliseconds to wait=u32 50) -> ()  [unwired: 1 out]
        n144 = call-poly <vilib>:"WPI_SolenoidSet.vi"("Value"=WPI_SolenoidValue."On", "SolenoidDevRef"=w362) -> ()  [unwired: 8 in, 2 out]
        n145 = call-poly <vilib>:"WPI_SolenoidSet.vi"("Value"=WPI_SolenoidValue."Off", "SolenoidDevRef"=w361) -> ()  [unwired: 8 in, 2 out]
        n146 = call <vilib>:"WPI_RobotDriveTankDrive.vi"("Right axis value"=w368, "Left axis value"=w369, "RobotDriveDevRef"=w371) -> ("Motor Values"=w366:dbl[], "RobotDriveDevRef"=w367:T5)  [unwired: 6 in, 1 out]
        n147 = call-poly <vilib>:"NT Write Value.vi"("Numeric Array"=w366, "Name"=w365) -> ()  [unwired: 9 in, 1 out]
      }
    }
    frame "middle delay" {
      # "Forward for 0 second"
      # "turn left for 0 seconds"
      # "Straight  for 0 seconds"
      # "forward for half a second"
      # "turn right"
      # "left for 1/4 of a second"
      # "forward for a second"
      # "eggstra step"
      # "forward for half a second"
      # "Delay 5 seconds"
      # "SHOOT THE CUBE"
      n148 = call <vilib>:"WPI_SolenoidRefNum Registry Get.vi"("refnum name"="Solenoid A.2") -> ("SolenoidDevRef"=w415:T11)  [unwired: 9 in, 1 out]
      n149 = call <vilib>:"WPI_SolenoidRefNum Registry Get.vi"("refnum name"="Solenoid A") -> ("SolenoidDevRef"=w413:T11)  [unwired: 9 in, 1 out]
      n150 = call <vilib>:"WPI_RobotDriveRefNum Registry Get.vi"("refnum name"="Left and Right Motors") -> ("RobotDriveDevRef"=w395:T5)  [unwired: 1 in, 9 out]
      n151 = for {
        N: 200 -> [_]
        tunnel: w395 -> [w496]
        tunnel: [w492] -> w396
        tunnel: "RobotDrive Motors" ("Name") -> [w490]
        tunnel: [w490] -> w397 mode=indexing
        tunnel: w413 -> [w489]
        tunnel: [w489] -> w414 mode=indexing
        tunnel: w415 -> [w488]
        tunnel: [w488] -> w416 mode=indexing
        w493 = 0.0  # RightSpeed
        w494 = 0.0  # LeftSpeed
        n152 = Wait (ms)(milliseconds to wait=u32 50) -> ()  [unwired: 1 out]
        n153 = call <vilib>:"WPI_RobotDriveTankDrive.vi"("Right axis value"=w493, "Left axis value"=w494, "RobotDriveDevRef"=w496) -> ("Motor Values"=w491:dbl[], "RobotDriveDevRef"=w492:T5)  [unwired: 6 in, 1 out]
        n154 = call-poly <vilib>:"NT Write Value.vi"("Numeric Array"=w491, "Name"=w490) -> ()  [unwired: 9 in, 1 out]
      }
      n155 = for {
        N: 45 -> [_]
        tunnel: w396 -> [w480]
        tunnel: [w484] -> w400 mode=indexing
        tunnel: w397 -> [w484] mode=indexing
        tunnel: w414 -> [w481] mode=indexing
        tunnel: w416 -> [w482] mode=indexing
        tunnel: [w481] -> w417 mode=indexing
        tunnel: [w482] -> w418 mode=indexing
        tunnel: [w483] -> w419 mode=indexing
        w485 = -0.65  # RightSpeed
        w486 = -0.65  # LeftSpeed
        n156 = Wait (ms)(milliseconds to wait=u32 50) -> ()  [unwired: 1 out]
        n157 = call <vilib>:"WPI_RobotDriveTankDrive.vi"("Right axis value"=w485, "Left axis value"=w486, "RobotDriveDevRef"=w480) -> ("Motor Values"=w479:dbl[], "RobotDriveDevRef"=w483:T5)  [unwired: 6 in, 1 out]
        n158 = call-poly <vilib>:"NT Write Value.vi"("Numeric Array"=w479, "Name"=w484) -> ()  [unwired: 9 in, 1 out]
      }
      n159 = for {
        N: 40 -> [_]
        tunnel: [w455] -> w399 mode=indexing
        tunnel: w400 -> [w456] mode=indexing
        tunnel: [w456] -> w398 mode=indexing
        tunnel: w417 -> [w457] mode=indexing
        tunnel: w418 -> [w459] mode=indexing
        tunnel: w419 -> [w458] mode=indexing
        w462 = 0.0  # RightSpeed
        w463 = 0.0  # LeftSpeed
        n160 = Wait (ms)(milliseconds to wait=u32 50) -> ()  [unwired: 1 out]
        n161 = call-poly <vilib>:"WPI_SolenoidSet.vi"("Value"=WPI_SolenoidValue."On", "SolenoidDevRef"=w457) -> ()  [unwired: 8 in, 2 out]
        n162 = call <vilib>:"WPI_RobotDriveTankDrive.vi"("Right axis value"=w462, "Left axis value"=w463, "RobotDriveDevRef"=w458) -> ("Motor Values"=w454:dbl[], "RobotDriveDevRef"=w455:T5)  [unwired: 6 in, 1 out]
        n163 = call-poly <vilib>:"NT Write Value.vi"("Numeric Array"=w454, "Name"=w456) -> ()  [unwired: 9 in, 1 out]
        n164 = call-poly <vilib>:"WPI_SolenoidSet.vi"("Value"=WPI_SolenoidValue."Off", "SolenoidDevRef"=w459) -> ()  [unwired: 8 in, 2 out]
      }
      n165 = for {
        N: 0 -> [_]
        tunnel: w399 -> [w478] mode=indexing
        tunnel: w398 -> [w473] mode=indexing
        tunnel: [w473] -> w401 mode=indexing
        tunnel: [w472] -> w402 mode=indexing
        w475 = -0.55  # RightSpeed
        w476 = -0.55  # LeftSpeed
        n166 = Wait (ms)(milliseconds to wait=u32 50) -> ()  [unwired: 1 out]
        n167 = call <vilib>:"WPI_RobotDriveTankDrive.vi"("Right axis value"=w475, "Left axis value"=w476, "RobotDriveDevRef"=w478) -> ("Motor Values"=w474:dbl[], "RobotDriveDevRef"=w472:T5)  [unwired: 6 in, 1 out]
        n168 = call-poly <vilib>:"NT Write Value.vi"("Numeric Array"=w474, "Name"=w473) -> ()  [unwired: 9 in, 1 out]
      }
      n169 = for {
        N: 0 -> [_]
        tunnel: w402 -> [w471] mode=indexing
        tunnel: [w468] -> w404 mode=indexing
        tunnel: w401 -> [w466] mode=indexing
        tunnel: [w466] -> w403 mode=indexing
        w465 = 0.8  # LeftSpeed
        w469 = -0.8  # RightSpeed
        n170 = Wait (ms)(milliseconds to wait=u32 50) -> ()  [unwired: 1 out]
        n171 = call <vilib>:"WPI_RobotDriveTankDrive.vi"("Right axis value"=w469, "Left axis value"=w465, "RobotDriveDevRef"=w471) -> ("Motor Values"=w467:dbl[], "RobotDriveDevRef"=w468:T5)  [unwired: 6 in, 1 out]
        n172 = call-poly <vilib>:"NT Write Value.vi"("Numeric Array"=w467, "Name"=w466) -> ()  [unwired: 9 in, 1 out]
      }
      n173 = for {
        N: 0 -> [_]
        tunnel: w404 -> [w453] mode=indexing
        tunnel: [w449] -> w406 mode=indexing
        tunnel: w403 -> [w447] mode=indexing
        tunnel: [w447] -> w405 mode=indexing
        w450 = -0.75  # RightSpeed
        w451 = -0.75  # LeftSpeed
        n174 = Wait (ms)(milliseconds to wait=u32 50) -> ()  [unwired: 1 out]
        n175 = call <vilib>:"WPI_RobotDriveTankDrive.vi"("Right axis value"=w450, "Left axis value"=w451, "RobotDriveDevRef"=w453) -> ("Motor Values"=w448:dbl[], "RobotDriveDevRef"=w449:T5)  [unwired: 6 in, 1 out]
        n176 = call-poly <vilib>:"NT Write Value.vi"("Numeric Array"=w448, "Name"=w447) -> ()  [unwired: 9 in, 1 out]
      }
      n177 = for {
        N: 40 -> [_]
        tunnel: w406 -> [w446] mode=indexing
        tunnel: [w443] -> w408 mode=indexing
        tunnel: w405 -> [w441] mode=indexing
        tunnel: [w441] -> w407 mode=indexing
        w444 = 0.0  # RightSpeed
        w445 = 0.0  # LeftSpeed
        (unwired) u32 50 ("milliseconds to wait")
        n178 = call <vilib>:"WPI_RobotDriveTankDrive.vi"("Right axis value"=w444, "Left axis value"=w445, "RobotDriveDevRef"=w446) -> ("Motor Values"=w442:dbl[], "RobotDriveDevRef"=w443:T5)  [unwired: 6 in, 1 out]
        n179 = call-poly <vilib>:"NT Write Value.vi"("Numeric Array"=w442, "Name"=w441) -> ()  [unwired: 9 in, 1 out]
      }
      n180 = for {
        N: 0 -> [_]
        tunnel: w408 -> [w440] mode=indexing
        tunnel: [w436] -> w410 mode=indexing
        tunnel: w407 -> [w434] mode=indexing
        tunnel: [w434] -> w409 mode=indexing
        w437 = -0.55  # RightSpeed
        w438 = 0.55  # LeftSpeed
        n181 = Wait (ms)(milliseconds to wait=u32 50) -> ()  [unwired: 1 out]
        n182 = call <vilib>:"WPI_RobotDriveTankDrive.vi"("Right axis value"=w437, "Left axis value"=w438, "RobotDriveDevRef"=w440) -> ("Motor Values"=w435:dbl[], "RobotDriveDevRef"=w436:T5)  [unwired: 6 in, 1 out]
        n183 = call-poly <vilib>:"NT Write Value.vi"("Numeric Array"=w435, "Name"=w434) -> ()  [unwired: 9 in, 1 out]
      }
      n184 = for {
        N: 0 -> [_]
        tunnel: w410 -> [w433] mode=indexing
        tunnel: [w429] -> w411 mode=indexing
        tunnel: w409 -> [w427] mode=indexing
        tunnel: [w427] -> w412 mode=indexing
        w430 = -0.7  # RightSpeed
        w431 = -0.7  # LeftSpeed
        n185 = Wait (ms)(milliseconds to wait=u32 50) -> ()  [unwired: 1 out]
        n186 = call <vilib>:"WPI_RobotDriveTankDrive.vi"("Right axis value"=w430, "Left axis value"=w431, "RobotDriveDevRef"=w433) -> ("Motor Values"=w428:dbl[], "RobotDriveDevRef"=w429:T5)  [unwired: 6 in, 1 out]
        n187 = call-poly <vilib>:"NT Write Value.vi"("Numeric Array"=w428, "Name"=w427) -> ()  [unwired: 9 in, 1 out]
      }
      n188 = for {
        N: 40 -> [_]
        tunnel: w411 -> [w426] mode=indexing
        tunnel: [w422] -> _ mode=indexing
        tunnel: w412 -> [w420] mode=indexing
        tunnel: [w420] -> _ mode=indexing
        w423 = 0.0  # RightSpeed
        w424 = 0.0  # LeftSpeed
        n189 = Wait (ms)(milliseconds to wait=u32 50) -> ()  [unwired: 1 out]
        n190 = call <vilib>:"WPI_RobotDriveTankDrive.vi"("Right axis value"=w423, "Left axis value"=w424, "RobotDriveDevRef"=w426) -> ("Motor Values"=w421:dbl[], "RobotDriveDevRef"=w422:T5)  [unwired: 6 in, 1 out]
        n191 = call-poly <vilib>:"NT Write Value.vi"("Numeric Array"=w421, "Name"=w420) -> ()  [unwired: 9 in, 1 out]
      }
    }
    frame "right delay" {
      # "Delay 5 seconds"
      # "Forward for 1 seconds"
      # "Turn left for 1 seconds"
      # "Forward for 4 seconds"
      # "Turn right  1 second"
      # "SHOOT THE CUBE"
      # "Forward 0.5 seconds"
      n192 = call <vilib>:"WPI_SolenoidRefNum Registry Get.vi"("refnum name"="Solenoid A.2") -> ("SolenoidDevRef"=w499:T11)  [unwired: 9 in, 1 out]
      n193 = call <vilib>:"WPI_SolenoidRefNum Registry Get.vi"("refnum name"="Solenoid A") -> ("SolenoidDevRef"=w505:T11)  [unwired: 9 in, 1 out]
      n194 = call <vilib>:"WPI_RobotDriveRefNum Registry Get.vi"("refnum name"="Left and Right Motors") -> ("RobotDriveDevRef"=w515:T5)  [unwired: 1 in, 9 out]
      n195 = for {
        N: 100 -> [_]
        tunnel: w515 -> [w543]
        tunnel: [w539] -> w514
        tunnel: [w537] -> w516 mode=indexing
        tunnel: "RobotDrive Motors" ("Name") -> [w537]
        tunnel: [w536] -> w506 mode=indexing
        tunnel: w505 -> [w536]
        tunnel: [w535] -> w500 mode=indexing
        tunnel: w499 -> [w535]
        w540 = 0.0  # RightSpeed
        w541 = 0.0  # LeftSpeed
        n196 = Wait (ms)(milliseconds to wait=u32 50) -> ()  [unwired: 1 out]
        n197 = call <vilib>:"WPI_RobotDriveTankDrive.vi"("Right axis value"=w540, "Left axis value"=w541, "RobotDriveDevRef"=w543) -> ("Motor Values"=w538:dbl[], "RobotDriveDevRef"=w539:T5)  [unwired: 6 in, 1 out]
        n198 = call-poly <vilib>:"NT Write Value.vi"("Numeric Array"=w538, "Name"=w537) -> ()  [unwired: 9 in, 1 out]
      }
      n199 = for {
        N: 10 -> [_]
        tunnel: w514 -> [w599]
        tunnel: [w595] -> w531
        tunnel: [w593] -> w530 mode=indexing
        tunnel: w516 -> [w593] mode=indexing
        tunnel: [w592] -> w507 mode=indexing
        tunnel: w506 -> [w592] mode=indexing
        tunnel: [w591] -> w501 mode=indexing
        tunnel: w500 -> [w591] mode=indexing
        w596 = -0.7  # RightSpeed
        w597 = -0.7  # LeftSpeed
        n200 = Wait (ms)(milliseconds to wait=u32 50) -> ()  [unwired: 1 out]
        n201 = call <vilib>:"WPI_RobotDriveTankDrive.vi"("Right axis value"=w596, "Left axis value"=w597, "RobotDriveDevRef"=w599) -> ("Motor Values"=w594:dbl[], "RobotDriveDevRef"=w595:T5)  [unwired: 6 in, 1 out]
        n202 = call-poly <vilib>:"NT Write Value.vi"("Numeric Array"=w594, "Name"=w593) -> ()  [unwired: 9 in, 1 out]
      }
      n203 = for {
        N: 30 -> [_]
        tunnel: w531 -> [w579]
        tunnel: [w575] -> w527
        tunnel: [w573] -> w528 mode=indexing
        tunnel: w530 -> [w573] mode=indexing
        tunnel: [w572] -> w508 mode=indexing
        tunnel: w507 -> [w572] mode=indexing
        tunnel: [w571] -> w502 mode=indexing
        tunnel: w501 -> [w571] mode=indexing
        w576 = 0.7  # RightSpeed
        w577 = -0.7  # LeftSpeed
        n204 = Wait (ms)(milliseconds to wait=u32 50) -> ()  [unwired: 1 out]
        n205 = call <vilib>:"WPI_RobotDriveTankDrive.vi"("Right axis value"=w576, "Left axis value"=w577, "RobotDriveDevRef"=w579) -> ("Motor Values"=w574:dbl[], "RobotDriveDevRef"=w575:T5)  [unwired: 6 in, 1 out]
        n206 = call-poly <vilib>:"NT Write Value.vi"("Numeric Array"=w574, "Name"=w573) -> ()  [unwired: 9 in, 1 out]
      }
      n207 = for {
        N: 600 -> [_]
        tunnel: w527 -> [w570]
        tunnel: [w566] -> w522 mode=indexing
        tunnel: w528 -> [w564] mode=indexing
        tunnel: [w564] -> w525 mode=indexing
        tunnel: [w563] -> w509 mode=indexing
        tunnel: w508 -> [w563] mode=indexing
        tunnel: [w562] -> w503 mode=indexing
        tunnel: w502 -> [w562] mode=indexing
        w567 = -0.9  # RightSpeed
        w568 = -0.9  # LeftSpeed
        n208 = Wait (ms)(milliseconds to wait=u32 50) -> ()  [unwired: 1 out]
        n209 = call <vilib>:"WPI_RobotDriveTankDrive.vi"("Right axis value"=w567, "Left axis value"=w568, "RobotDriveDevRef"=w570) -> ("Motor Values"=w565:dbl[], "RobotDriveDevRef"=w566:T5)  [unwired: 6 in, 1 out]
        n210 = call-poly <vilib>:"NT Write Value.vi"("Numeric Array"=w565, "Name"=w564) -> ()  [unwired: 9 in, 1 out]
      }
      n211 = for {
        N: 20 -> [_]
        tunnel: w522 -> [w561] mode=indexing
        tunnel: [w557] -> w521 mode=indexing
        tunnel: w525 -> [w555] mode=indexing
        tunnel: [w555] -> w524 mode=indexing
        tunnel: [w554] -> w510 mode=indexing
        tunnel: w509 -> [w554] mode=indexing
        tunnel: [w553] -> w504 mode=indexing
        tunnel: w503 -> [w553] mode=indexing
        w558 = -0.5  # RightSpeed
        w559 = 0.5  # LeftSpeed
        n212 = Wait (ms)(milliseconds to wait=u32 50) -> ()  [unwired: 1 out]
        n213 = call <vilib>:"WPI_RobotDriveTankDrive.vi"("Right axis value"=w558, "Left axis value"=w559, "RobotDriveDevRef"=w561) -> ("Motor Values"=w556:dbl[], "RobotDriveDevRef"=w557:T5)  [unwired: 6 in, 1 out]
        n214 = call-poly <vilib>:"NT Write Value.vi"("Numeric Array"=w556, "Name"=w555) -> ()  [unwired: 9 in, 1 out]
      }
      n215 = for {
        N: 110 -> [_]
        tunnel: w521 -> [w552] mode=indexing
        tunnel: [w548] -> w520 mode=indexing
        tunnel: w524 -> [w546] mode=indexing
        tunnel: [w546] -> w523 mode=indexing
        tunnel: w510 -> [w545] mode=indexing
        tunnel: w504 -> [w544] mode=indexing
        tunnel: [w545] -> w498 mode=indexing
        tunnel: [w544] -> w497 mode=indexing
        w549 = -0.8  # RightSpeed
        w550 = -0.8  # LeftSpeed
        n216 = Wait (ms)(milliseconds to wait=u32 50) -> ()  [unwired: 1 out]
        n217 = call <vilib>:"WPI_RobotDriveTankDrive.vi"("Right axis value"=w549, "Left axis value"=w550, "RobotDriveDevRef"=w552) -> ("Motor Values"=w547:dbl[], "RobotDriveDevRef"=w548:T5)  [unwired: 6 in, 1 out]
        n218 = call-poly <vilib>:"NT Write Value.vi"("Numeric Array"=w547, "Name"=w546) -> ()  [unwired: 9 in, 1 out]
      }
      n219 = for {
        N: 40 -> [_]
        tunnel: w520 -> [w590] mode=indexing
        tunnel: [w586] -> _
        tunnel: [w584] -> _ mode=indexing
        tunnel: w523 -> [w584] mode=indexing
        tunnel: w498 -> [w581] mode=indexing
        tunnel: w497 -> [w580] mode=indexing
        w587 = 0.0  # RightSpeed
        w588 = 0.0  # LeftSpeed
        n220 = Wait (ms)(milliseconds to wait=u32 50) -> ()  [unwired: 1 out]
        n221 = call-poly <vilib>:"WPI_SolenoidSet.vi"("Value"=WPI_SolenoidValue."On", "SolenoidDevRef"=w581) -> ()  [unwired: 8 in, 2 out]
        n222 = call-poly <vilib>:"WPI_SolenoidSet.vi"("Value"=WPI_SolenoidValue."Off", "SolenoidDevRef"=w580) -> ()  [unwired: 8 in, 2 out]
        n223 = call <vilib>:"WPI_RobotDriveTankDrive.vi"("Right axis value"=w587, "Left axis value"=w588, "RobotDriveDevRef"=w590) -> ("Motor Values"=w585:dbl[], "RobotDriveDevRef"=w586:T5)  [unwired: 6 in, 1 out]
        n224 = call-poly <vilib>:"NT Write Value.vi"("Numeric Array"=w585, "Name"=w584) -> ()  [unwired: 9 in, 1 out]
      }
    }
    frame "extra" {
      # "SHOOT THE CUBE"
      n225 = call <vilib>:"WPI_SolenoidRefNum Registry Get.vi"("refnum name"="Solenoid A.2") -> ("SolenoidDevRef"=w635:T11)  [unwired: 9 in, 1 out]
      n226 = call <vilib>:"WPI_SolenoidRefNum Registry Get.vi"("refnum name"="Solenoid A") -> ("SolenoidDevRef"=w629:T11)  [unwired: 9 in, 1 out]
      n227 = call <vilib>:"WPI_RobotDriveRefNum Registry Get.vi"("refnum name"="Left and Right Motors") -> ("RobotDriveDevRef"=w622:T5)  [unwired: 1 in, 9 out]
      n228 = for {
        N: 200 -> [_]
        tunnel: w622 -> [w646]
        tunnel: [w642] -> w623
        tunnel: [w640] -> w621 mode=indexing
        tunnel: "RobotDrive Motors" ("Name") -> [w640]
        tunnel: [w639] -> w628 mode=indexing
        tunnel: w629 -> [w639]
        tunnel: [w638] -> w634 mode=indexing
        tunnel: w635 -> [w638]
        w643 = 0.0  # RightSpeed
        w644 = 0.0  # LeftSpeed
        n229 = Wait (ms)(milliseconds to wait=u32 50) -> ()  [unwired: 1 out]
        n230 = call <vilib>:"WPI_RobotDriveTankDrive.vi"("Right axis value"=w643, "Left axis value"=w644, "RobotDriveDevRef"=w646) -> ("Motor Values"=w641:dbl[], "RobotDriveDevRef"=w642:T5)  [unwired: 6 in, 1 out]
        n231 = call-poly <vilib>:"NT Write Value.vi"("Numeric Array"=w641, "Name"=w640) -> ()  [unwired: 9 in, 1 out]
      }
      n232 = for {
        N: 10 -> [_]
        tunnel: w623 -> [w702]
        tunnel: [w698] -> w611
        tunnel: [w696] -> w612 mode=indexing
        tunnel: w621 -> [w696] mode=indexing
        tunnel: [w695] -> w627 mode=indexing
        tunnel: w628 -> [w695] mode=indexing
        tunnel: [w694] -> w633 mode=indexing
        tunnel: w634 -> [w694] mode=indexing
        w699 = -0.7  # RightSpeed
        w700 = -0.7  # LeftSpeed
        n233 = Wait (ms)(milliseconds to wait=u32 50) -> ()  [unwired: 1 out]
        n234 = call <vilib>:"WPI_RobotDriveTankDrive.vi"("Right axis value"=w699, "Left axis value"=w700, "RobotDriveDevRef"=w702) -> ("Motor Values"=w697:dbl[], "RobotDriveDevRef"=w698:T5)  [unwired: 6 in, 1 out]
        n235 = call-poly <vilib>:"NT Write Value.vi"("Numeric Array"=w697, "Name"=w696) -> ()  [unwired: 9 in, 1 out]
      }
      n236 = for {
        N: 30 -> [_]
        tunnel: w611 -> [w682]
        tunnel: [w678] -> w614
        tunnel: [w676] -> w613 mode=indexing
        tunnel: w612 -> [w676] mode=indexing
        tunnel: [w675] -> w626 mode=indexing
        tunnel: w627 -> [w675] mode=indexing
        tunnel: [w674] -> w632 mode=indexing
        tunnel: w633 -> [w674] mode=indexing
        w679 = -0.7  # RightSpeed
        w680 = 0.7  # LeftSpeed
        n237 = Wait (ms)(milliseconds to wait=u32 50) -> ()  [unwired: 1 out]
        n238 = call <vilib>:"WPI_RobotDriveTankDrive.vi"("Right axis value"=w679, "Left axis value"=w680, "RobotDriveDevRef"=w682) -> ("Motor Values"=w677:dbl[], "RobotDriveDevRef"=w678:T5)  [unwired: 6 in, 1 out]
        n239 = call-poly <vilib>:"NT Write Value.vi"("Numeric Array"=w677, "Name"=w676) -> ()  [unwired: 9 in, 1 out]
      }
      n240 = for {
        N: 600 -> [_]
        tunnel: w614 -> [w673]
        tunnel: [w669] -> w618 mode=indexing
        tunnel: w613 -> [w667] mode=indexing
        tunnel: [w667] -> w615 mode=indexing
        tunnel: [w666] -> w625 mode=indexing
        tunnel: w626 -> [w666] mode=indexing
        tunnel: [w665] -> w631 mode=indexing
        tunnel: w632 -> [w665] mode=indexing
        w670 = -0.9  # RightSpeed
        w671 = -0.9  # LeftSpeed
        n241 = Wait (ms)(milliseconds to wait=u32 50) -> ()  [unwired: 1 out]
        n242 = call <vilib>:"WPI_RobotDriveTankDrive.vi"("Right axis value"=w670, "Left axis value"=w671, "RobotDriveDevRef"=w673) -> ("Motor Values"=w668:dbl[], "RobotDriveDevRef"=w669:T5)  [unwired: 6 in, 1 out]
        n243 = call-poly <vilib>:"NT Write Value.vi"("Numeric Array"=w668, "Name"=w667) -> ()  [unwired: 9 in, 1 out]
      }
      n244 = for {
        N: 20 -> [_]
        tunnel: w618 -> [w664] mode=indexing
        tunnel: [w660] -> w619 mode=indexing
        tunnel: w615 -> [w658] mode=indexing
        tunnel: [w658] -> w616 mode=indexing
        tunnel: [w657] -> w624 mode=indexing
        tunnel: w625 -> [w657] mode=indexing
        tunnel: [w656] -> w630 mode=indexing
        tunnel: w631 -> [w656] mode=indexing
        w661 = 0.5  # RightSpeed
        w662 = -0.5  # LeftSpeed
        n245 = Wait (ms)(milliseconds to wait=u32 50) -> ()  [unwired: 1 out]
        n246 = call <vilib>:"WPI_RobotDriveTankDrive.vi"("Right axis value"=w661, "Left axis value"=w662, "RobotDriveDevRef"=w664) -> ("Motor Values"=w659:dbl[], "RobotDriveDevRef"=w660:T5)  [unwired: 6 in, 1 out]
        n247 = call-poly <vilib>:"NT Write Value.vi"("Numeric Array"=w659, "Name"=w658) -> ()  [unwired: 9 in, 1 out]
      }
      n248 = for {
        N: 100 -> [_]
        tunnel: w619 -> [w655] mode=indexing
        tunnel: [w651] -> w620 mode=indexing
        tunnel: w616 -> [w649] mode=indexing
        tunnel: [w649] -> w617 mode=indexing
        tunnel: w624 -> [w648] mode=indexing
        tunnel: w630 -> [w647] mode=indexing
        tunnel: [w648] -> w636 mode=indexing
        tunnel: [w647] -> w637 mode=indexing
        w652 = -0.8  # RightSpeed
        w653 = -0.8  # LeftSpeed
        n249 = Wait (ms)(milliseconds to wait=u32 50) -> ()  [unwired: 1 out]
        n250 = call <vilib>:"WPI_RobotDriveTankDrive.vi"("Right axis value"=w652, "Left axis value"=w653, "RobotDriveDevRef"=w655) -> ("Motor Values"=w650:dbl[], "RobotDriveDevRef"=w651:T5)  [unwired: 6 in, 1 out]
        n251 = call-poly <vilib>:"NT Write Value.vi"("Numeric Array"=w650, "Name"=w649) -> ()  [unwired: 9 in, 1 out]
      }
      n252 = for {
        N: 40 -> [_]
        tunnel: w620 -> [w693] mode=indexing
        tunnel: [w689] -> _
        tunnel: [w687] -> _ mode=indexing
        tunnel: w617 -> [w687] mode=indexing
        tunnel: w636 -> [w684] mode=indexing
        tunnel: w637 -> [w683] mode=indexing
        w690 = 0.0  # RightSpeed
        w691 = 0.0  # LeftSpeed
        n253 = Wait (ms)(milliseconds to wait=u32 50) -> ()  [unwired: 1 out]
        n254 = call-poly <vilib>:"WPI_SolenoidSet.vi"("Value"=WPI_SolenoidValue."On", "SolenoidDevRef"=w684) -> ()  [unwired: 8 in, 2 out]
        n255 = call-poly <vilib>:"WPI_SolenoidSet.vi"("Value"=WPI_SolenoidValue."Off", "SolenoidDevRef"=w683) -> ()  [unwired: 8 in, 2 out]
        n256 = call <vilib>:"WPI_RobotDriveTankDrive.vi"("Right axis value"=w690, "Left axis value"=w691, "RobotDriveDevRef"=w693) -> ("Motor Values"=w688:dbl[], "RobotDriveDevRef"=w689:T5)  [unwired: 6 in, 1 out]
        n257 = call-poly <vilib>:"NT Write Value.vi"("Numeric Array"=w688, "Name"=w687) -> ()  [unwired: 9 in, 1 out]
      }
    }
  }
  n258 = call <vilib>:"WPI_JoystickRefNum Registry Get.vi"("refnum name"="Joystick 1") -> ("JoystickDevRef"=w8:T2)  [unwired: 1 in, 9 out]
  n259 = call <vilib>:"WPI_JoystickGetValues.vi"("JoystickDevRef"=w8) -> ("Axes"=w6:dbl[])  [unwired: 6 in, 4 out]
  n260 = Index Array(array=w6, index=2) -> ()  [unwired: 1 out]
  n261 = call-poly <vilib>:"NT Write Value.vi"("Numeric Array"=w6, "Name"="Joystick 1/Axes") -> ()  [unwired: 9 in, 1 out]
